vi "NI VeriStand - Open Multiple Waveforms Write Session (CDB).vi"(7 "Communication Properties":T1, 8 "error in (no error)":errorcluster, 10 "dt":dbl=nan, 11 "CDB Waveform Data References":T2[](array[typedef])) -> (0 "error out":errorcluster, 3 "Multiple Waveforms Write Session (CDB)":refnum<class "Multiple Waveforms Write (CDB).lvclass">)   [LabVIEW 2020, in "NI_VS Custom Device Waveform API.lvlib" / "Multiple Waveforms Write (CDB).lvclass"]
doc: "Opens a session for reading data from or writing data to a specific waveform or waveforms associated with a custom device. You must manually select the instance to use according to the number of waveforms with which you want to interact, whether the data type of the waveforms is DBL or CDB, and whether you want to read or write waveform data."
uses:
  Multiple Waveforms Write (CDB).lvclass
  D:/p4/penguin/lvaddon/Veristand/master/src/LabVIEW/vilib/NI VeriStand/Custom Device Waveform API/Waveform Session.lvclass
  Custom Device API/Waveform Data Reference.ctl
  Communication Properties.ctl
  Internal Comm Classes/WPL Comm/WPL Comm (2D CDB)/WPL Comm (2D CDB).lvclass
  Access mode.ctl
  Multiple Waveforms Write (CDB).lvclass/Multiple Waveforms Write (CDB).ctl
  Waveform Session.lvclass/Waveform Session.ctl
  Waveform Session.lvclass
  NI_VS Custom Device Waveform API.lvlib
  Custom Device API/Custom Device API.lvlib
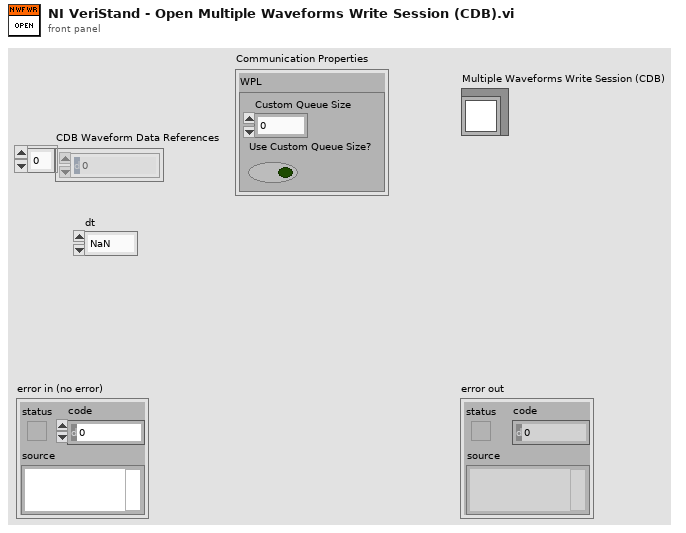
[diagram p1: front panel]
types:
  T1 = typedef "NI_VS Custom Device Waveform API.lvlib/Communication Properties.ctl" = cluster{"WPL":cluster{"Custom Queue Size":i32, "Use Custom Queue Size?":bool}}
  T2 = typedef "Custom Device API.lvlib/Waveform Data Reference.ctl" = i32
  T3 = typedef "NI_VS Custom Device Waveform API.lvlib/Access mode.ctl" = enum16{"Read", "Write"}
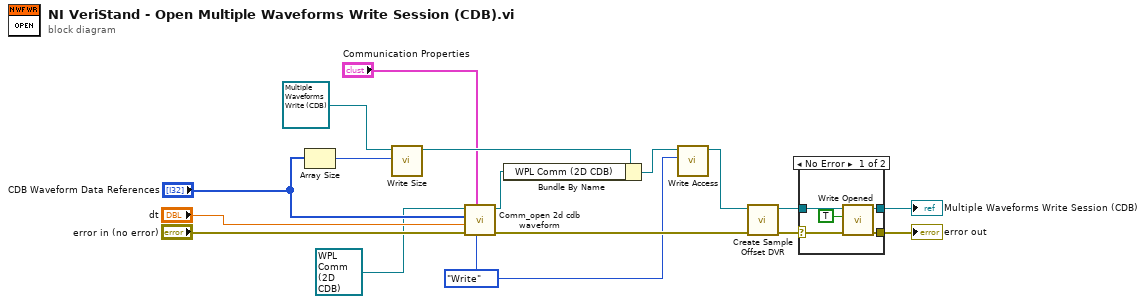
[diagram p0: block diagram]
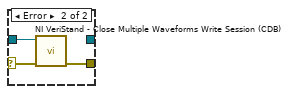
[diagram p2: hidden frame]
diagram:
  w8 = Access_mode."Write" ("Access")
  n1 = Array Size(array="CDB Waveform Data References") -> (size(s)=w9:i32)
  n2 = call "Write Size.vi"("Size"=w9, "Waveform Session in"=refnum<class "Multiple Waveforms Write (CDB).lvclass"> refnum ("Waveform API.lvlib:2D DBL Write.lvclass")) -> ("Waveform Session out"=w4:refnum<class "Multiple Waveforms Write (CDB).lvclass">)  [unwired: 9 in]
  n3 = call "Comm_open 2d cdb waveform.vi"("Access"=w8, "Communication Properties"="Communication Properties", "error in (no error)"="error in (no error)", "dt"="dt", "Waveform Data References"="CDB Waveform Data References", "WPL Comm (2D CDB) in"=refnum<class "WPL Comm (2D CDB).lvclass"> refnum ("Internal Comm Classes.lvlib:WPL Comm (2D CDB).lvclass")) -> ("error out"=w13:errorcluster, "WPL Comm (2D CDB) out"=w3:refnum<class "WPL Comm (2D CDB).lvclass">)  [unwired: 4 in]
  n4 = Bundle By Name(cluster=w4, "WPL Comm (2D CDB)"=w3) -> (w2:refnum<class "Multiple Waveforms Write (CDB).lvclass">)
  n5 = call "Write Access.vi"("Access"=w8, "Waveform Session in"=w2) -> ("Waveform Session out"=w7:refnum<class "Multiple Waveforms Write (CDB).lvclass">)  [unwired: 9 in]
  n6 = call "Create Sample Offset DVR.vi"("error in (no error)"=w13, "Waveform Session in"=w7) -> ("error out"=w11:errorcluster, "Waveform Session out"=w12:refnum<class "Multiple Waveforms Write (CDB).lvclass">)  [unwired: 8 in]
  n7 = case shown="No Error" w11 {
    selector: w11 -> [w21 w24]
    tunnel: [w21 w23] -> w17
    tunnel: w12 -> [w20 w22]
    tunnel: [w19 _] -> w14
    frame No Error {
      n8 = call "Write Opened.vi"("Opened"=TRUE, "Waveform Session in"=w20) -> ("Waveform Session out"=w19:refnum<class "Multiple Waveforms Write (CDB).lvclass">)  [unwired: 9 in]
    }
    frame Error {
      n9 = call "NI VeriStand - Close Multiple Waveforms Write Session (CDB).vi"("error in (no error)"=w24, "Multiple Waveforms Write Session (CDB)"=w22) -> ("error out"=w23:errorcluster)  [unwired: 9 in]
    }
  }
  "error out" <- w17
  "Multiple Waveforms Write Session (CDB)" <- w14
